vi "IN RANGE LOGIC.vi"() -> ()   [LabVIEW 2017]
uses:
  <userlib>/_OpenG.lib/array/array.llb/Sort 1D Array (DBL)__ogtk.vi
panel:
  out "sorted array":dbl[](array[numeric])
  out "TRIP RESET\nACHIVED":bool
  out "TRIP RESET\nHIGHER FAIL":bool
  out "TRIP RESET\nLOWER FAIL":bool
  out "TRIP FORCE\nHIGHER FAIL":bool
  out "TRIP FORCE\nLOWER FAIL":bool
  in  "RESULT":bool
  in  "Y":dbl format="%#_13g"
  in  "X":dbl format="%#_13g"
  in  "Boolean":bool
  in  "stop":bool
  out "XY Graph":cluster{"X DISTANCE":dbl[], "Y LOAD":dbl[]}(graph) caption="XY Graph - Dark"
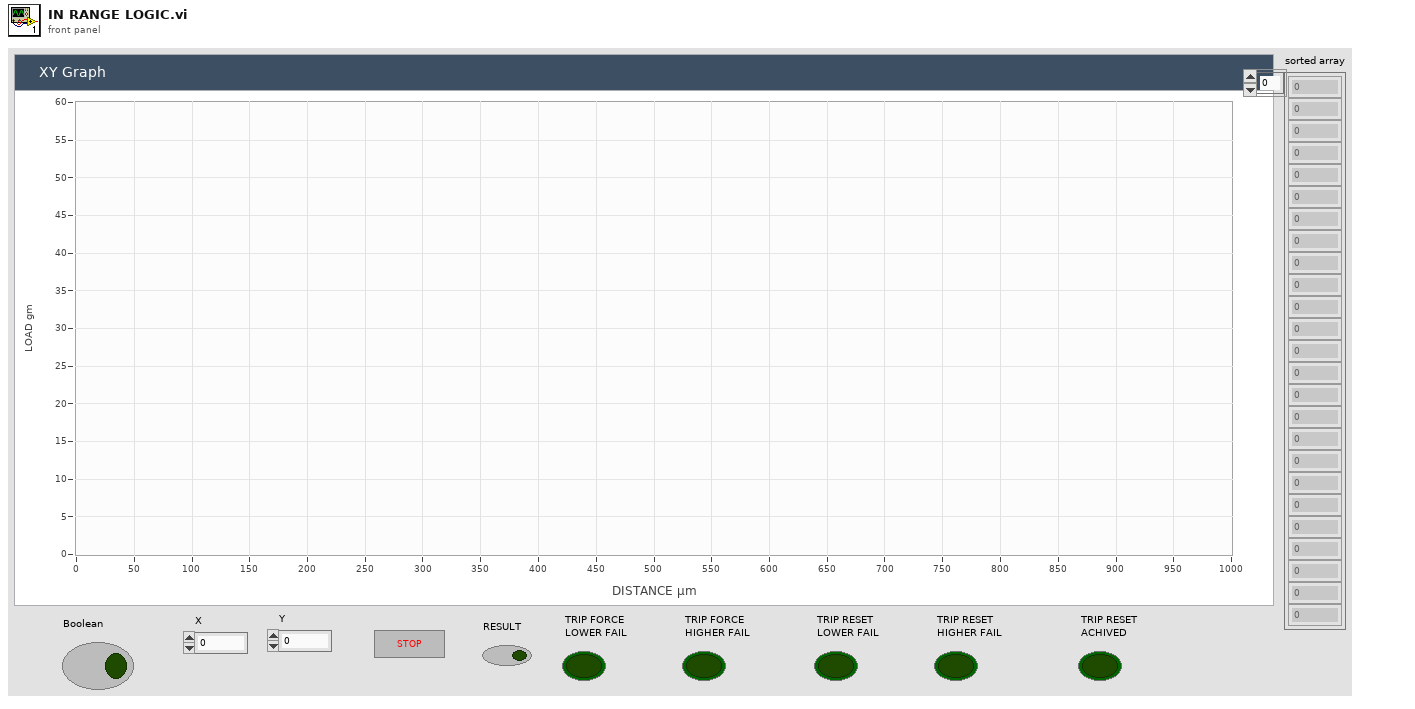
[diagram p1: front panel]
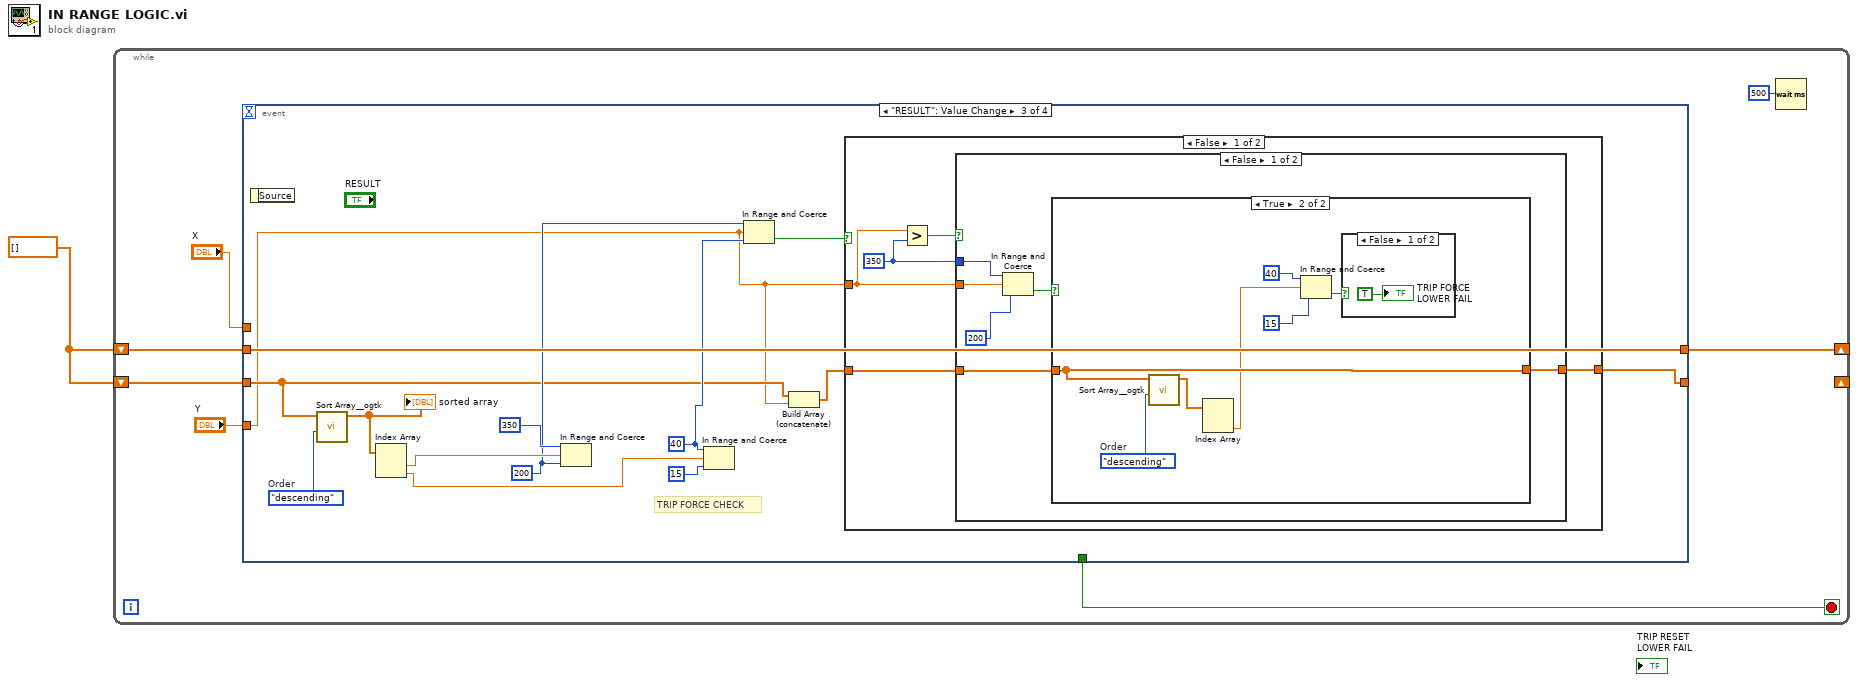
[diagram p0: block diagram]
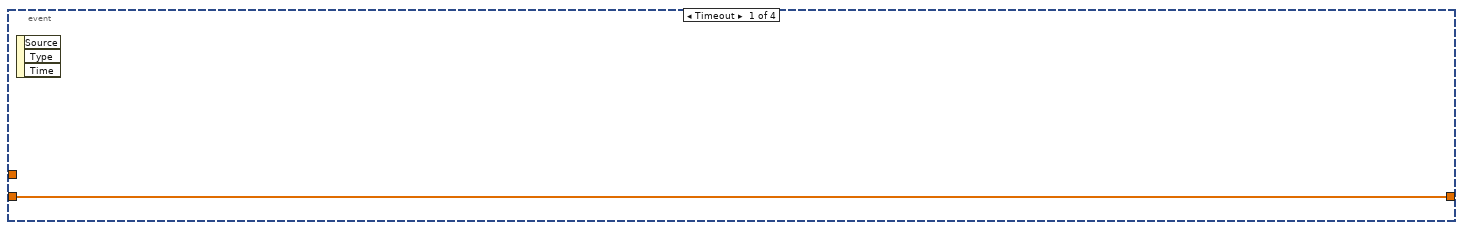
[diagram p2: hidden frame]
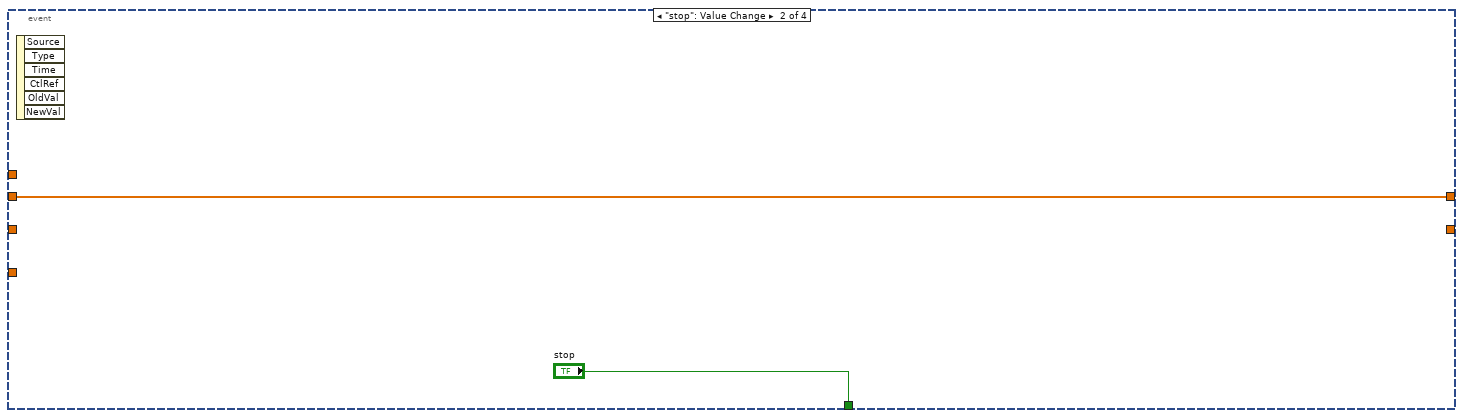
[diagram p3: hidden frame]
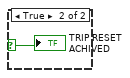
[diagram p5: hidden frame]
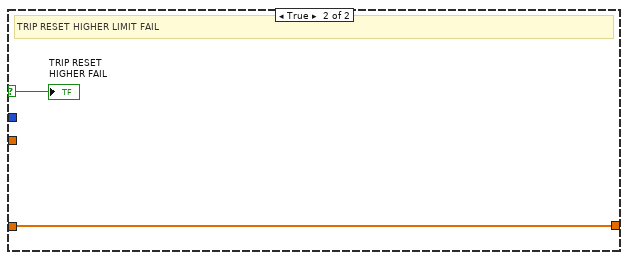
[diagram p6: hidden frame]
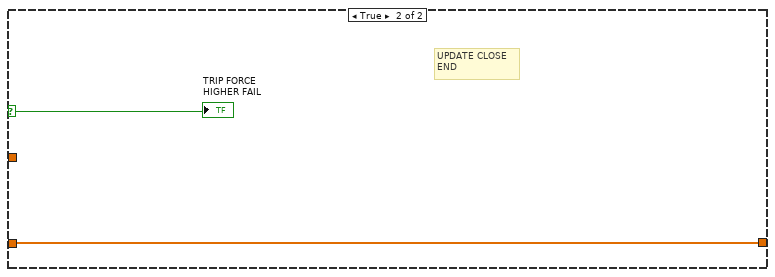
[diagram p7: hidden frame]
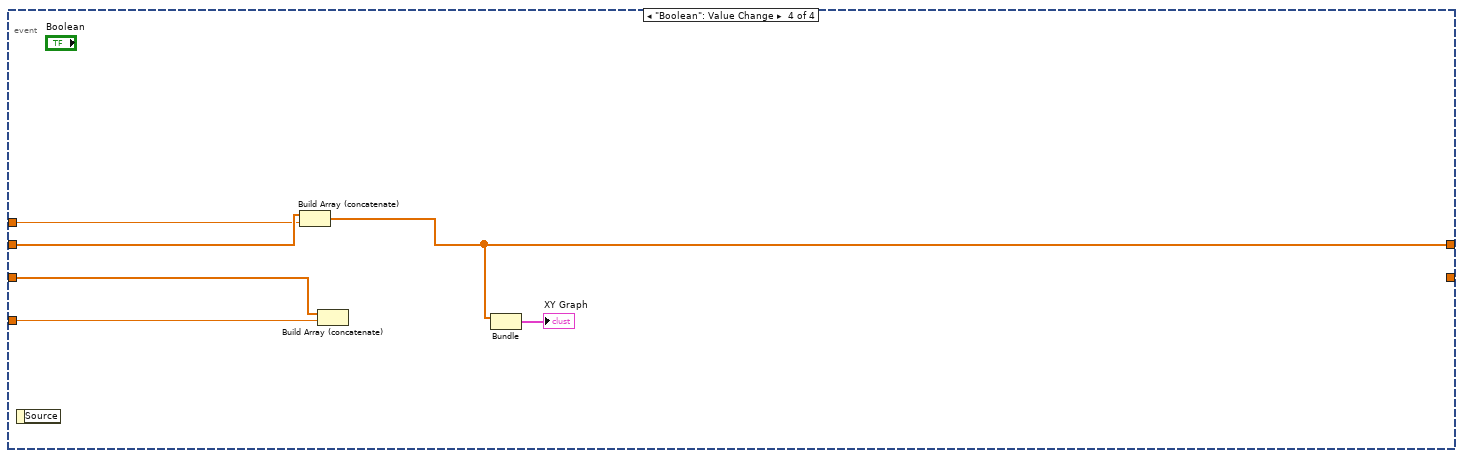
[diagram p8: hidden frame]
diagram:
  w1 = dbl[] []
  n1 = while {
    shift-right: [w7] -> _
    shift-left: w1 -> [w6]
    shift-right: _ -> [_]
    shift-left: w1 -> [w5]
    stop <- w4 stop-if-true
    n2 = event shown="[2] \"RESULT\": Value Change" {
      selector: _ -> [_ _ _ _]
      dyn-events: _ -> [_ _ _ _]
      timeout: _ -> [_ _ _ _]
      tunnel: [w9 w10 w25 w53] -> w7
      tunnel: w6 -> [w9 w10 w25 w54]
      tunnel: [_ _ w15 _] -> _
      tunnel: w5 -> [_ _ w14 w55]
      tunnel: [_ "stop" _ _] -> w4
      tunnel: "X" -> [_ _ _ w52]
      tunnel: "Y" -> [_ _ w12 w51]
      event Timeout {
        n3 = event-data() -> ()  [unwired: 1 in, 3 out]
      }
      event "stop": Value Change {
        n4 = event-data() -> ()  [unwired: 1 in, 6 out]
      }
      event "RESULT": Value Change {
        w17 = 40
        w20 = enum16{"ascending", "descending"}."descending"  # Order
        w18 = 200
        # "TRIP FORCE CHECK"
        n5 = event-data() -> ()  [unwired: 1 in, 1 out]
        n6 = call-poly <userlib>:"Sort Array__ogtk.vi"("Order"=w20, "Array in"=w14) -> ("Sorted Array out"=w21:dbl[])  [unwired: 8 in, 1 out]
        "sorted array" <- w21
        n7 = Index Array(array=w21) -> (element #1=w23:dbl, element #2=w22:dbl)  [unwired: 2 in]
        n8 = In Range and Coerce(upper limit=350, x=w23, lower limit=w18) -> ()  [unwired: 2 out]
        n9 = In Range and Coerce(upper limit=w17, x=w22, lower limit=15) -> ()  [unwired: 2 out]
        n10 = In Range and Coerce(upper limit=w18, x=w12, lower limit=w17) -> (In Range?=w16:bool)  [unwired: 1 out]
        n11 = Build Array (concatenate)(w14, w12) -> (w13:dbl[])
        n12 = case shown="False" w16 {
          selector: w16 -> [_ w50]
          tunnel: w12 -> [w30 _]
          tunnel: w13 -> [w27 w49]
          tunnel: [w26 w49] -> w15
          frame False {
            w29 = 350
            n13 = Greater?(x=w30, y=w29) -> (0:w28:bool)
            n14 = case shown="False" w28 {
              selector: w28 -> [_ w48]
              tunnel: w30 -> [w32 _]
              tunnel: w29 -> [w34 _]
              tunnel: w27 -> [w33 w47]
              tunnel: [w31 w47] -> w26
              frame False {
                n15 = In Range and Coerce(upper limit=w34, x=w32, lower limit=200) -> (In Range?=w35:bool)  [unwired: 1 out]
                n16 = case shown="True" w35 {
                  tunnel: w33 -> [w37 w42]
                  tunnel: [w37 w42] -> w31
                  frame False {
                  }
                  frame True {
                    w41 = enum16{"ascending", "descending"}."descending"  # Order
                    n17 = call-poly <userlib>:"Sort Array__ogtk.vi"("Order"=w41, "Array in"=w42) -> ("Sorted Array out"=w40:dbl[])  [unwired: 8 in, 1 out]
                    n18 = Index Array(array=w40) -> (element #2=w39:dbl)  [unwired: 2 in, 1 out]
                    n19 = In Range and Coerce(upper limit=40, x=w39, lower limit=15) -> (In Range?=w38:bool)  [unwired: 1 out]
                    n20 = case shown="False" w38 {
                      selector: w38 -> [_ w46]
                      frame False {
                        "TRIP FORCE\nLOWER FAIL" <- TRUE
                      }
                      frame True {
                        "TRIP RESET\nACHIVED" <- w46
                      }
                    }
                  }
                }
              }
              frame True {
                # "TRIP RESET HIGHER LIMIT FAIL"
                "TRIP RESET\nHIGHER FAIL" <- w48
              }
            }
          }
          frame True {
            # "UPDATE CLOSE\nEND"
            "TRIP FORCE\nHIGHER FAIL" <- w50
          }
        }
      }
      event "Boolean": Value Change {
        n21 = event-data() -> ()  [unwired: 1 in, 1 out]
        n22 = Build Array (concatenate)(w54, w52) -> (w53:dbl[])
        n23 = Build Array (concatenate)(w55, w51) -> ()  [unwired: 1 out]
        n24 = Bundle(w53) -> (→"XY Graph":cluster{dbl[], void})  [unwired: 2 in]
      }
    }
    n25 = Wait (ms)(milliseconds to wait=500) -> ()  [unwired: 1 out]
  }
